vi "popup-mark-frame.vi"(6 "frame.name":string, 8 "error in (no error)":errorcluster, 10 "frame.type.in":T1) -> (0 "error out":errorcluster, 2 "grame.type.out":T1, 4 "ok 2":bool)   [LabVIEW 2015]
uses:
  subs/frame.type.ctl
  controls/frame-actions.ctl
panel:
  in  "cancel":bool
  in  "ok":bool
  in  "frame.type":T1 caption="this is a test"
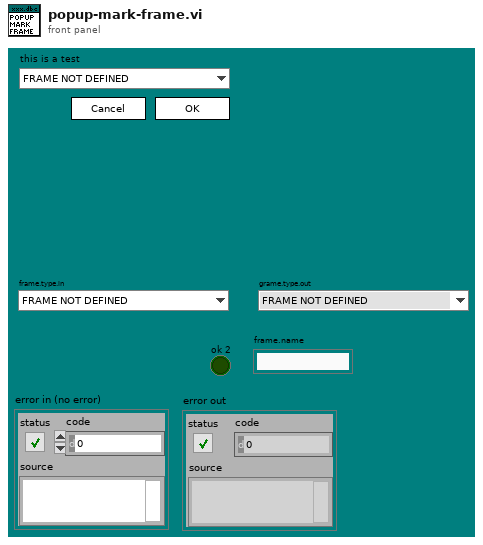
[diagram p1: front panel]
types:
  T1 = typedef "frame.type.ctl" = enum16{"FRAME NOT DEFINED", "DUT OUTPUT FRAME", "DUT INPUT FRAME"}
  T2 = typedef "frame-actions.ctl" = enum32{"frame.mdf", "input.frame", "output.frame", "unmark", "exit"}
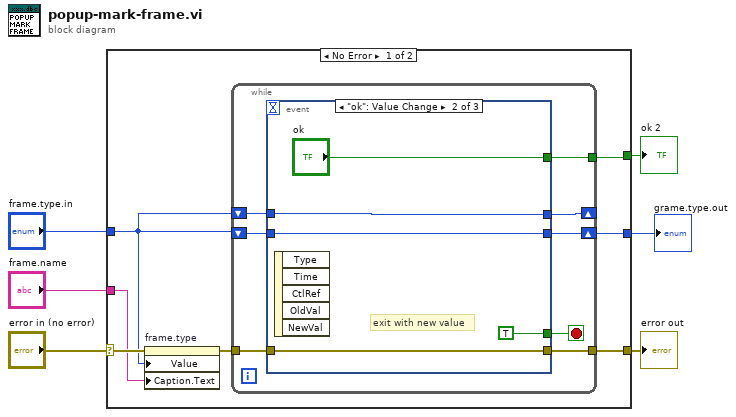
[diagram p0: block diagram]
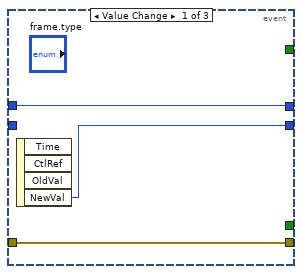
[diagram p2: hidden frame]
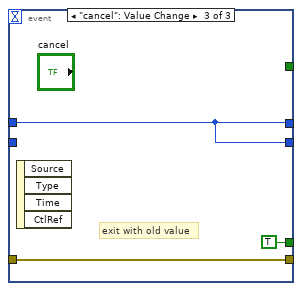
[diagram p3: hidden frame]
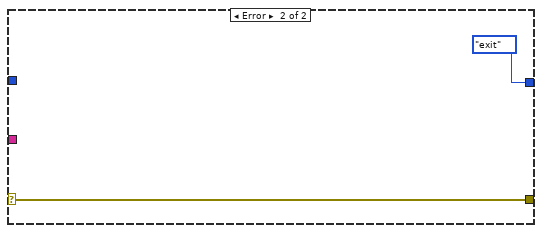
[diagram p4: hidden frame]
diagram:
  n1 = case shown="No Error" "error in (no error)" {
    selector: "error in (no error)" -> [w12 w34]
    tunnel: [w13 w34] -> w5
    tunnel: "frame.type.in" -> [w8 _]
    tunnel: [w10 frame-actions."exit" ("symbol")] -> w3
    tunnel: "frame.name" -> [w9 _]
    tunnel: [w7 _] -> w1
    frame No Error {
      n2 = property on="frame.type" class="Enum (strict)"(error in=w12, "Value"=w8, "Caption.Text"=w9) -> (error out=w11:errorcluster)  [unwired: 1 in, 1 out]
      n3 = while {
        tunnel: w11 -> [w21]
        tunnel: [w20] -> w13
        shift-right: [w19] -> w10
        shift-left: w8 -> [w18]
        shift-right: [w16] -> _
        shift-left: w8 -> [w15]
        tunnel: [w14] -> w7
        stop <- w17 stop-if-true
        n4 = event shown="[1] \"ok\": Value Change" {
          selector: _ -> [_ _ _]
          dyn-events: _ -> [_ _ _]
          timeout: _ -> [_ _ _]
          tunnel: w21 -> [w24 w28 w32]
          tunnel: [w24 w28 w32] -> w20
          tunnel: [w23 w27 w30] -> w19
          tunnel: w18 -> [_ w27 _]
          tunnel: [_ TRUE TRUE] -> w17
          tunnel: [w22 w26 w30] -> w16
          tunnel: w15 -> [w22 w26 w30]
          tunnel: [_ "ok" _] -> w14
          event Value Change {
            n5 = event-data() -> ("NewVal"=w23:T1)  [unwired: 1 in, 3 out]
          }
          event "ok": Value Change {
            # "exit with new value"
            n6 = event-data() -> ()  [unwired: 1 in, 5 out]
          }
          event "cancel": Value Change {
            # "exit with old value"
            n7 = event-data() -> ()  [unwired: 1 in, 4 out]
          }
        }
      }
    }
    frame Error {
    }
  }
  "error out" <- w5
  "grame.type.out" <- w3
  "ok 2" <- w1
